vi "TEST_TestContoller.vi"() -> ()   [LabVIEW 2024]
uses:
  Control Definitions/Def_PumpSpeed.ctl
  Control Definitions/DEF_CalConstants.ctl
  Control Definitions/DEF_PumpCtlRefs.ctl
  Control Definitions/Def CalTable.ctl
  Control Definitions/Def CalCoef.ctl
  Control Definitions/Def_LevelCalCoef.ctl
  Control Definitions/Def_Status18v7.ctl
  Control Definitions/DEF_TestInfo.ctl
  Control Definitions/Def TestState.ctl
  Control Definitions/Registry Keys.ctl
  Control Definitions/Def Results3.ctl
  Control Definitions/Def_ATPStatus.ctl
  Control Definitions/Global 2.vi
  Control Definitions/Global 1.vi
panel:
  out "TEST State Out":T1
  in  "Sim":bool=TRUE
  out "Test Info":T2={"Job Number"="", "Unit Number"="", "Serial Number"="", "Technician Name"="", "Calibration Date"="Cal Date", "Calibrator"="Cal by", "Calibration Slope"="M", "Calibration Offset"="B", "Config File Name"="Cal Date"}
  out "Pump Out":T4
  out "Cal Coef":T5={"Level"={"M"=-0.9990777034816695, "B"=9.617362923679963, "Mc"=-1.0009231479344565, "Bc"=9.626241172397878, "LMe"=7.844}, "Dataq Ch"=[{"B"=-0.34241100677002123, "M"=175.4094780519764}, {"B"=-0.7865736704446391, "M"=174.89102005231038}]}
  in  "Default Cal Table":T7={"Level"={"LSf"=2.6, "LMf"=3.511, "LKf"=6.112, "LMe"=7.844, "LKe"=1.775, "LSe"=8.0}, "DataQ CH"=[{"RqLA"=0.577, "RmLA"=102.9, "RqHA"=5.052, "RmHA"=904.4}, {"RqLA"=0.577, "RmLA"=101.1, "RqHA"=5.116, "RmHA"=903.4}]}
  in  "End Prog":bool=TRUE
  out "Test Index Out":i32
  out "PumpCtlRef out":T8
  out "Reg Cal Constants":T9={"Measure High"="", "Laser High"="", "Measure Low"="", "Laser Low"="", "Cal Name"="", "Cal Date"="9/24/2024 9:21:12 AM", "Empty Inches"=8.0, "Full Inches"=2.6, "Valid"=FALSE}
  in  "Pump Speed":T10
  in  "SimPV":bool
  out "Root Path":path=path "C:/AllenProjects/PWC-OLS"
  out "Time(ms)":dbl=1249.4499999994114
  out "Level":bool=TRUE
  out "DataQ":bool=TRUE
  in  "ChA":dbl(slide)=24.489795918367346 scale=0.0..1200.0
  in  "ChB":dbl(slide)=36.73469387755102 scale=0.0..1200.0
  in  "ChB +100":bool
  in  "ChA +100":bool
  in  "Check":bool
  out "Laser (raw)":dbl=1.9040000438690186 format="%#_4g"
  in  "DUT":i16=1
  in  "Pump JOG":bool=TRUE
  in  "Run Test":bool
  in  "Normal":cluster{u32, u32}[](array[cluster])=[{16711680, 1244948}]
  out "Level \nStatus":bool=TRUE
  out "DataQ\nStatus":bool=TRUE
  in  "Level SP":dbl(slide)=8.0 scale=8.5..2.0
  in  "Level PV":dbl(slide)=7.715118932422306 scale=8.5..2.0
  out "Level":dbl=7.715118932422306 format="%.3f"
  in  "Drain":bool
  in  "Fill":bool
  out "TEST Name":string="OLR001--cal"
  out "Time Stamp":timestamp=timestamp(3810639016.2712703 s since 1904-01-01)
  in  "stop":bool
  out "ChB Ohms":dbl=100.0340857774357 format="%.1f"
  out "ChA Ohms":dbl=100.79497115454612 format="%.1f"
  # "Calibration & Scaling Table\n               Tank         Key          Ref\n               Scale        Level        Measure\nEmpty\n\n\nFull"
  # "8.0      1.7752      7.844\n\n2.6      6.112        3.511"
  # "CHA             Resistance     Fill     Resistance   Drain"
  # "CHB           Resistance     Fill     Resistance   Drain"
  # "Simulated Resistor In"
  # "PUMP"
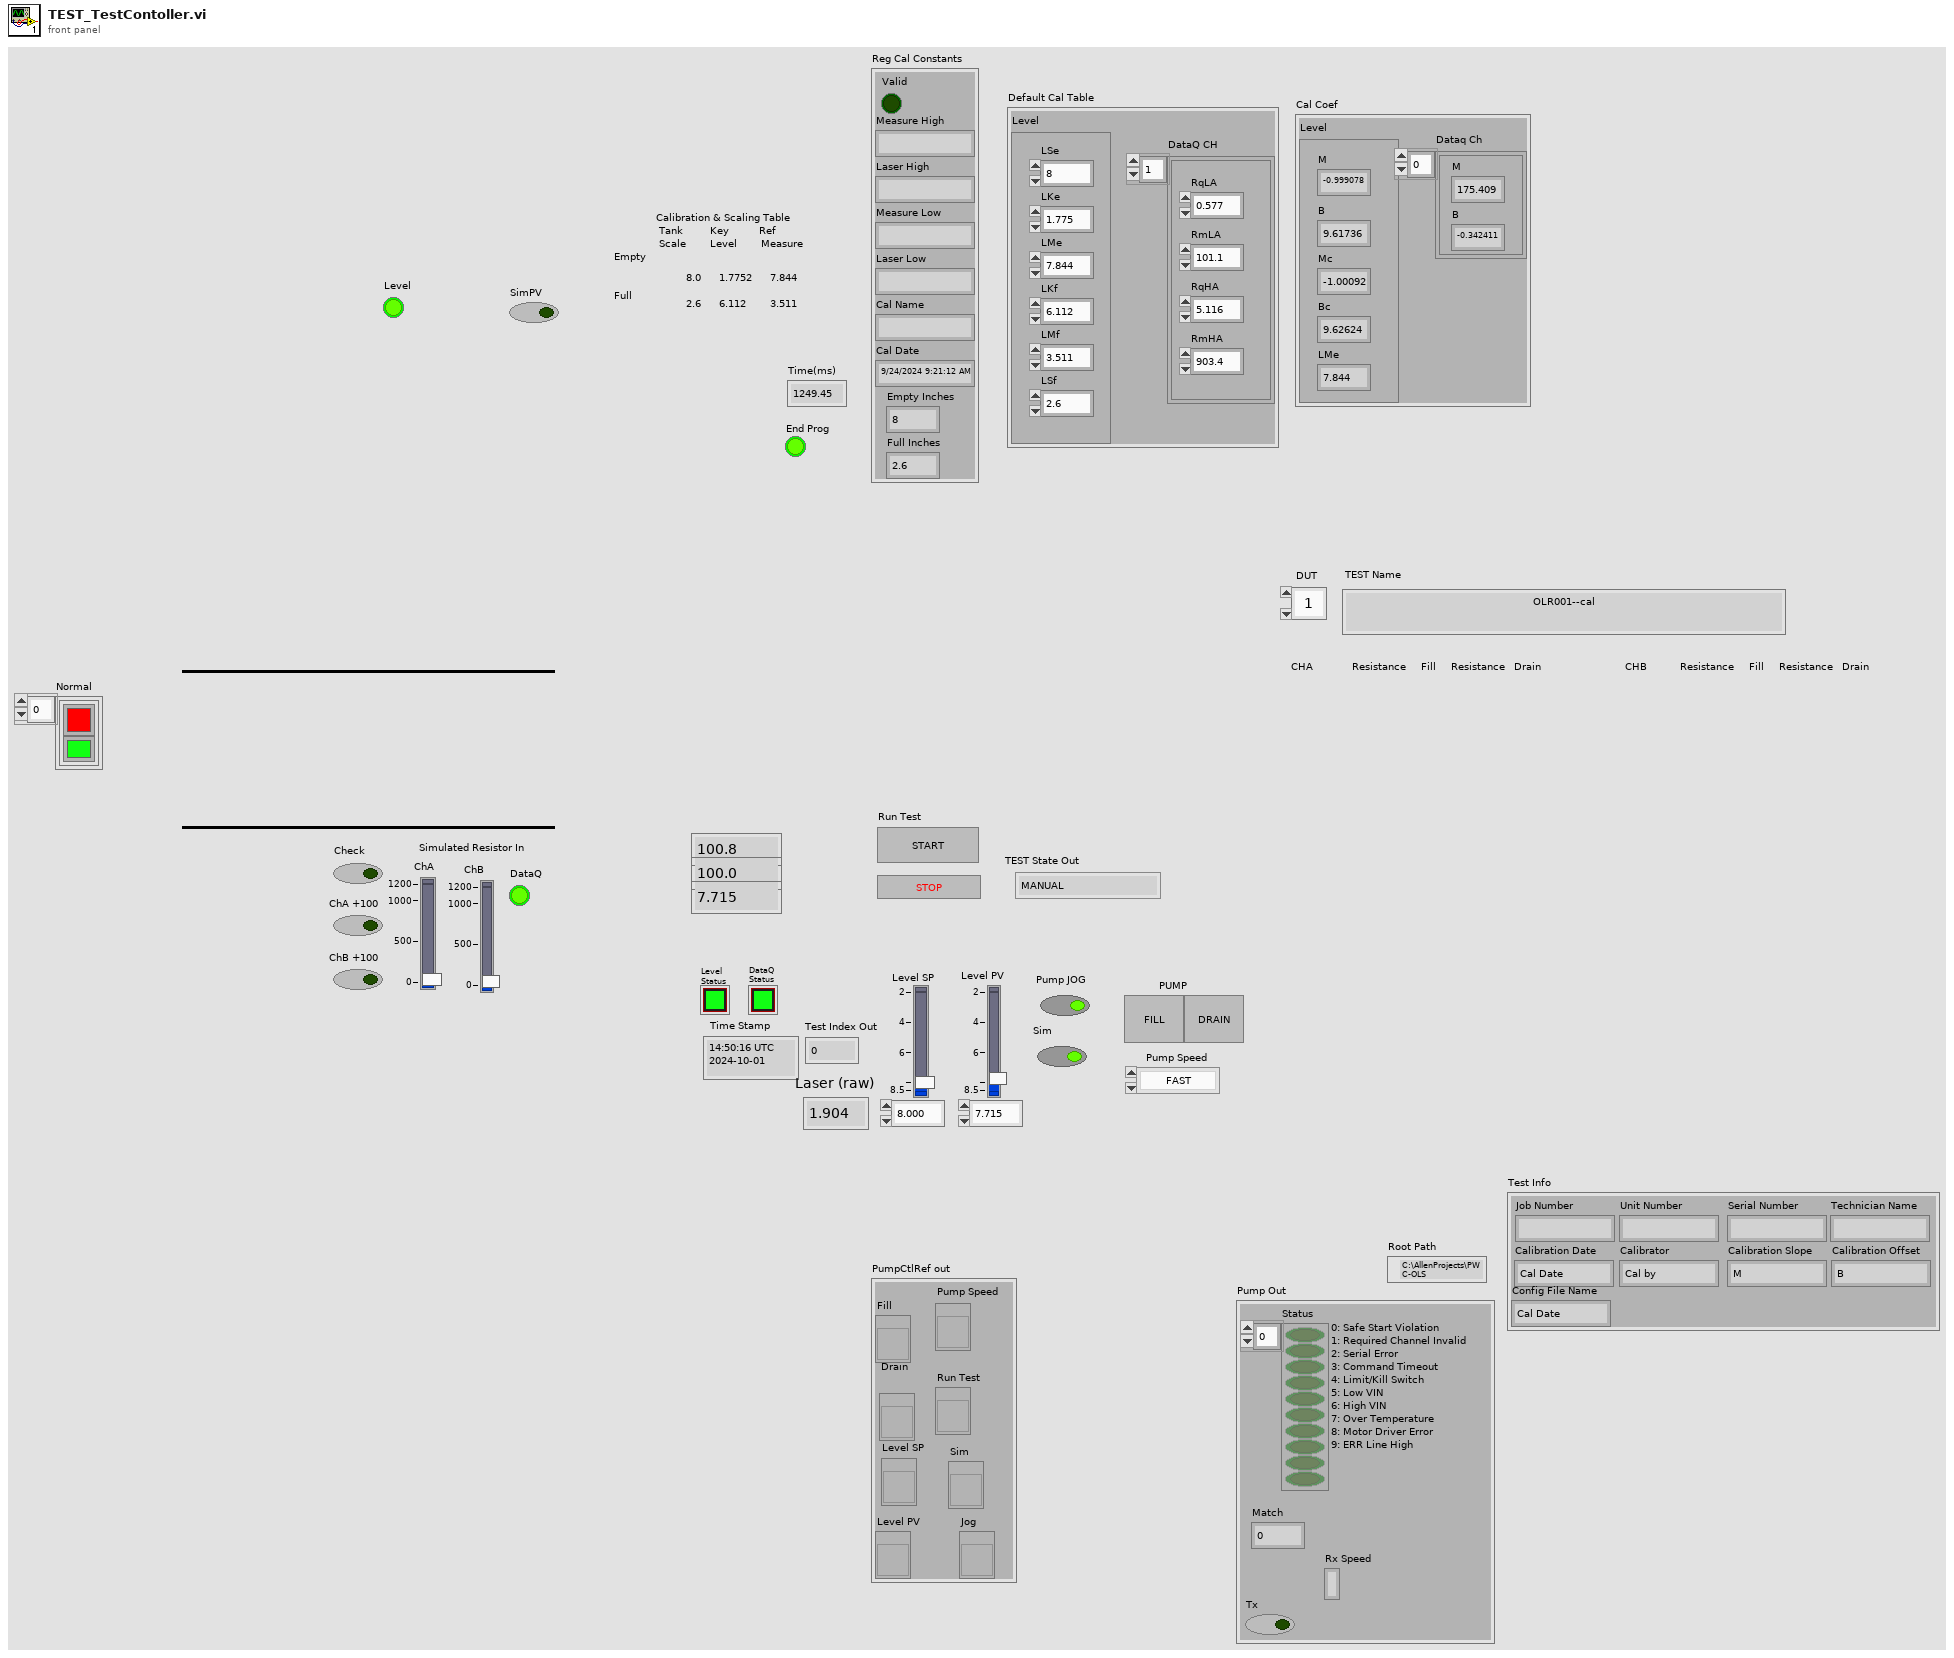
[diagram p1: front panel]
types:
  T1 = typedef "Def TestState.ctl" = enum16{"MANUAL", "Start", "Pre-Fill", "Pre-Fill Measure", "Pre-Drain", "Pre-Drain Measure", "Init-Record", "Load Fill Spec", "Filling Hi", "Wait1", "Record Fill", "Load Drain Spec", "Draining Lo", "Wait2", "Record Drain", "Empty", "Done"}
  T2 = typedef "DEF_TestInfo.ctl" = cluster{"Job Number":string, "Unit Number":string, "Serial Number":string, "Technician Name":string, "Calibration Date":string, "Calibrator":string, "Calibration Slope":string, "Calibration Offset":string, "Config File Name":string}
  T3 = typedef "Def_Status18v7.ctl" = bool[]
  T4 = cluster{"Status":T3, "Match":i32, "Rx Speed":string, "Tx":bool}
  T5 = typedef "Def CalCoef.ctl" = cluster{"Level":T6, "Dataq Ch":cluster{"B":dbl, "M":dbl}[]}
  T6 = typedef "Def_LevelCalCoef.ctl" = cluster{"M":dbl, "B":dbl, "Mc":dbl, "Bc":dbl, "LMe":dbl}
  T7 = typedef "Def CalTable.ctl" = cluster{"Level":cluster{"LSf":dbl, "LMf":dbl, "LKf":dbl, "LMe":dbl, "LKe":dbl, "LSe":dbl}, "DataQ CH":cluster{"RqLA":dbl, "RmLA":dbl, "RqHA":dbl, "RmHA":dbl}[]}
  T8 = typedef "DEF_PumpCtlRefs.ctl" = cluster{"Fill ":refnum<vi>, "Drain":refnum<vi>, "Level PV":refnum<vi>, "Pump Speed":refnum<vi>, "Run Test":refnum<vi>, "Sim":refnum<vi>, "Jog":refnum<vi>, "Level SP":refnum<vi>}
  T9 = typedef "DEF_CalConstants.ctl" = cluster{"Measure High":string, "Laser High":string, "Measure Low":string, "Laser Low":string, "Cal Name":string, "Cal Date":string, "Empty Inches":dbl, "Full Inches":dbl, "Valid":bool}
  T10 = typedef "Def_PumpSpeed.ctl" = enum16{"FAST", "SLOW", "CREEP", "STOP"}
  T11 = typedef "DEF_DataqParams.ctl" = cluster{"Visa Name":string, "Num Chan":i32, "Cal Coef":cluster{"M":dbl, "B":dbl}[], "Scale ":i32, "Cal Date":string, "Cal Technicain":string}
  T12 = typedef "DEF_18v7DriverInputs.ctl" = cluster{"Fill!Drain":bool, "Speed":i16, "Send Msg":bool, "Write Buf":string}
  T13 = typedef "Registry Keys.ctl" = enum16{"Report Files Key", "Config Files Key"}
  T14 = cluster{"Level \nStatus":refnum<vi>, "DataQ\nStatus":refnum<vi>}
  T15 = typedef "DEF_FullConfig.ctl" = cluster{"Bench Params":T16, "Test Params":dbl[][], "Pump Params":T17, "DataQ Params":T11, "Pump Control Ref":T8, "Bench Status":T18}
  T16 = typedef "DEF_BenchParams.ctl" = cluster{"Relative Root Name":string, "Values":cluster{"Step Levels":dbl, "Resistor Tolerence":dbl, "Sample Rate":dbl, "Resistor":dbl, "Wait Time":dbl}, "Report Template path":path, "Test Type":string, "Config File Name":string, "Config 2 Use":string, "Skip Pre Lube":bool}
  T17 = typedef "DEF_PumpParams.ctl" = cluster{"Empty Inches":dbl, "Full Inches":dbl, "RNG_SLOW":dbl, "RNG_CREEP":dbl, "RNG_STOP ":dbl, "VISA resource name":refnum<visa-resource-name>, "SPD_SLOW":i32, "SPD_CREEP":i32, "SPD_FAST":i32, "Zero template":path, "zero  Settle sec":i32, "Laser Slope":sgl, "Laser Offset":sgl, "Sim Fill Rate":sgl, "Cal Date":string, "Cal Technician":string}
  T18 = typedef "DEF_BenchStatus.ctl" = cluster{"Pump Status":refnum<vi>, "Instrumnet\n Status":refnum<vi>}
  T19 = typedef "Def Results3.ctl" = cluster{"Fill":dbl, "Status":T20, "Resistor":dbl, "Drain":dbl, "Resistor 2":dbl}
  T20 = typedef "Def_ATPStatus.ctl" = i16
  T21 = enum16{"MANUAL", "Start", "Filling", "FULL", "Draining", "EMPTY", "Done"}
  T22 = typedef "DEF_LevelOut.ctl" = cluster{"Laser ":cluster{"Raw":sgl, "Scaled":dbl}, "Level PV":dbl, "Fill":bool, "Drain":bool}
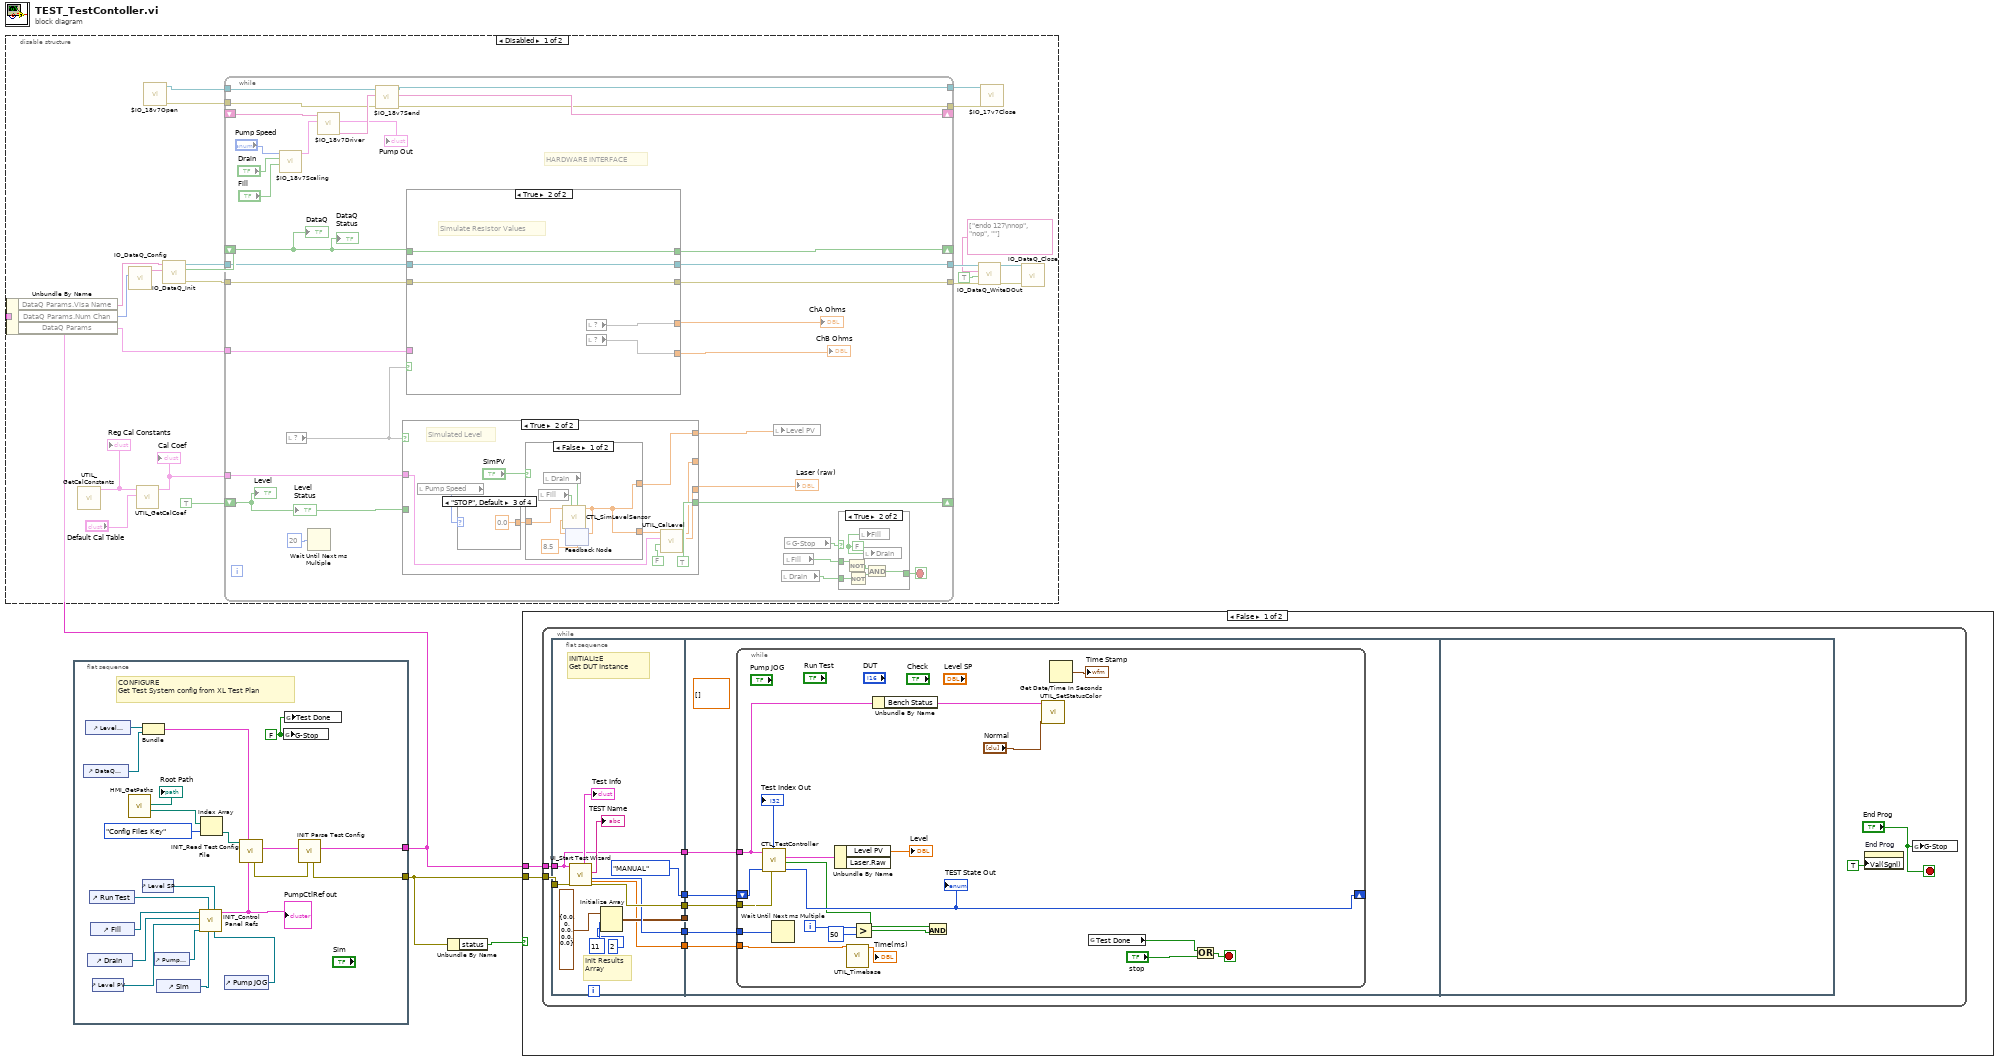
[diagram p0: block diagram]
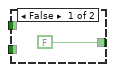
[diagram p2: hidden frame]
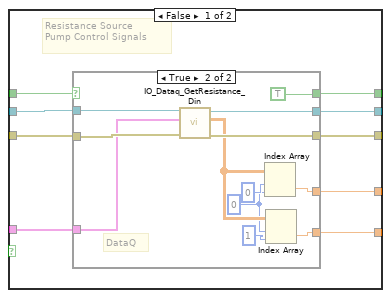
[diagram p3: hidden frame]
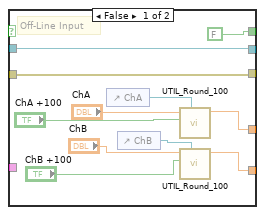
[diagram p4: hidden frame]
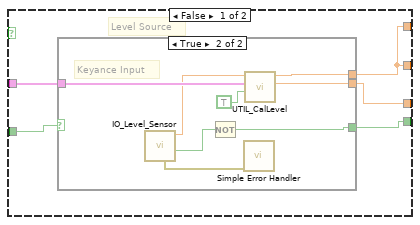
[diagram p5: hidden frame]
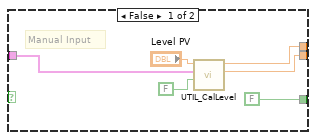
[diagram p6: hidden frame]
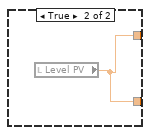
[diagram p7: hidden frame]
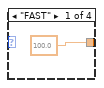
[diagram p8: hidden frame]
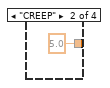
[diagram p9: hidden frame]
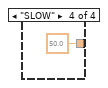
[diagram p10: hidden frame]
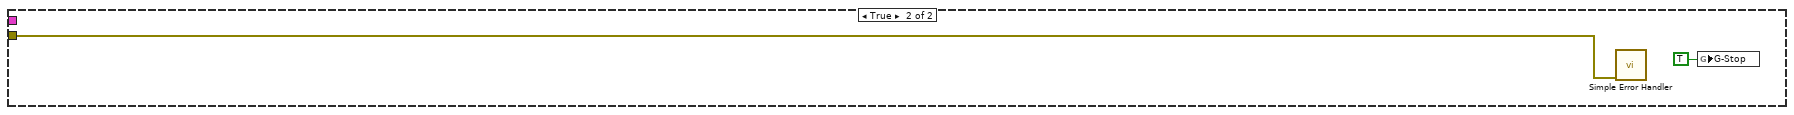
[diagram p12: hidden frame]
diagram:
  n1 = disable-structure shown="Disabled" {
    disable-tunnel: w1 -> [w4 _]
    frame Disabled {
      n2 = Unbundle By Name(w4) -> ("DataQ Params.Visa Name"=w6:string, "DataQ Params.Num Chan"=w7:i32, "DataQ Params"=w5:T11)
      n3 = call "UTIL_GetCalConstants.vi"() -> ("Cal Constants"=w14:T9)  [unwired: 10 in, 1 out]
      "Reg Cal Constants" <- w14
      n4 = call "IO_DataQ_Config.vi"("Num Chan"=w7) -> ("Init Message"=w25:string[])  [unwired: 10 in]
      n5 = call "UTIL_GetCalCoef.vi"("Cal Table"="Default Cal Table", "Cal Constants"=w14) -> ("Cal Coef"=w12:T5)  [unwired: 9 in]
      "Cal Coef" <- w12
      n6 = call "$IO_18v7Open.vi"() -> ("error out"=w11:errorcluster, "VISA Refnum out"=w10:refnum<visa-resource-name>)  [unwired: 10 in]
      n7 = call "IO_DataQ_Init.vi"("Command\nList"=w25, "RunTime VISA name"=w6) -> ("error out"=w23:errorcluster, "Connected?"=w22:bool, "VISA resource name out"=w24:refnum<visa-resource-name>)  [unwired: 7 in]
      n8 = while {
        shift-right: [w54] -> _
        shift-left: TRUE ("Pump \nStatus") -> [w41]
        tunnel: w24 -> [w53]
        tunnel: w23 -> [w52]
        tunnel: [w50] -> w20
        tunnel: [w51] -> w18
        shift-right: [w49] -> _
        shift-left: w22 -> [w48]
        tunnel: w12 -> [w26]
        shift-right: [w39] -> _
        shift-left: _ -> [w38]
        tunnel: w11 -> [w32]
        tunnel: w10 -> [w31]
        tunnel: [w30] -> w9
        tunnel: [w29] -> w8
        tunnel: w5 -> [w27]
        stop <- w45 stop-if-true
        # "HARDWARE INTERFACE"
        n9 = call "$IO_18v7Scaling.vi"("Drain"="Fill", "Fill"="Drain", "Pump Speed"="Pump Speed") -> ("Driver Signals"=w34:T12)  [unwired: 7 in, 1 out]
        n10 = local read item#-1() -> (w47)
        n11 = Wait Until Next ms Multiple(millisecond multiple=u32 20) -> ()  [unwired: 1 out]
        n12 = call "$IO_18v7Driver.vi"("Inputs"=w34, "Reply In"=w38) -> ("Tx Buf Out"=w33:string, "Outputs"=→"Pump Out":T4)  [unwired: 8 in]
        n13 = call "$IO_18v7Send.vi"("error in (no error)"=w32, "Tx Buf Out"=w33, "VISA Refnum in"=w31) -> ("error out"=w29:errorcluster, "read buffer"=w39:string, "VISA Refnum out"=w30:refnum<visa-resource-name>)  [unwired: 6 in]
        n14 = case shown="True" w47 {
          tunnel: [w102 w127] -> _
          tunnel: [w106 w129] -> w55
          tunnel: [w103 TRUE] -> w54
          tunnel: w41 -> [w105 _]
          tunnel: w26 -> [w104 w122]
          tunnel: [w102 w121] -> w40
          frame False {
            # "Level Source"
            n15 = case shown="True" w105 {
              tunnel: [w110 w113] -> w102
              tunnel: [w109 w118] -> w106
              tunnel: [FALSE ("status") w117] -> w103
              tunnel: w104 -> [w111 w119]
              frame False {
                # "Manual Input"
                n16 = call "UTIL_CalLevel.vi"("Key is In?"=FALSE, "Cal Coef"=w111, "Input"="Level PV") -> ("PVc"=w109:dbl, "PVs"=w110:dbl)  [unwired: 7 in]
              }
              frame True {
                # "Keyance Input"
                n17 = call "IO_Level_Sensor.vi"() -> ("status"=w115:bool, "PV (raw)"=w116:dbl, "error OUT"=w114:errorcluster)  [unwired: 9 in]
                n18 = Not(x=w115) -> (.not. x?=w117:bool)
                n19 = call <vilib>:"Simple Error Handler.vi"("error in (no error)"=w114) -> ()  [unwired: 4 in, 5 out]
                n20 = call "UTIL_CalLevel.vi"("Key is In?"=TRUE, "Cal Coef"=w119, "Input"=w116) -> ("PVc"=w118:dbl, "PVs"=w113:dbl)  [unwired: 7 in]
              }
            }
          }
          frame True {
            # "Simulated Level"
            n21 = local read "Pump Speed"() -> (w125:T10)
            n22 = case shown="\"STOP\", Default" w125 {
              tunnel: [100.0 ("Ctl Sig") 5.0 ("Ctl Sig") 0.0 ("Ctl Sig") 50.0 ("Ctl Sig")] -> w126
              frame "FAST" {
              }
              frame "CREEP" {
              }
              frame "STOP", Default {
              }
              frame "SLOW" {
              }
            }
            n23 = case shown="False" "SimPV" {
              tunnel: w126 -> [w135 _]
              tunnel: [w131 w137] -> w124
              tunnel: [w131 w137] -> w121
              frame False {
                n24 = local read "Fill"() -> (w136:bool)
                n25 = local read "Drain"() -> (w132:bool)
                n26 = feedback #1(8.5 ("PV Level Inch")) -> (w133:dbl)
                n27 = call "CTL_SimLevelSensor.vi"("Drain IN"=w132, "Fill IN"=w136, "Level PV in"=w133, "Pump Speed"=w135) -> ("PV Level Inch"=w131:dbl)  [unwired: 7 in]
                n28 = feedback-in #1(w131) -> ()
              }
              frame True {
                n29 = local read "Level PV"() -> (w137:dbl)
              }
            }
            n30 = call "UTIL_CalLevel.vi"("Key is In?"=FALSE, "Cal Coef"=w122, "Input"=w124) -> ("PVc"=w129:dbl, "PVs"=w127:dbl)  [unwired: 7 in]
          }
        }
        "Laser (raw)" <- w55
        n31 = case shown="True" w47 {
          tunnel: [w73 w98] -> w56
          tunnel: [w72 w97] -> w42
          tunnel: w53 -> [w66 w100]
          tunnel: w52 -> [w67 w99]
          tunnel: [w71 w99] -> w51
          tunnel: [w70 w100] -> w50
          tunnel: [w69 w101] -> w49
          tunnel: w48 -> [w68 w101]
          tunnel: w27 -> [w65 _]
          frame False {
            # "Resistance Source\nPump Control Signals"
            n32 = case shown="True" w68 {
              tunnel: [w77 w93] -> w73
              tunnel: [w78 w90] -> w72
              tunnel: [w79 w96] -> w70
              tunnel: [w80 w95] -> w71
              tunnel: [FALSE TRUE] -> w69
              tunnel: w67 -> [w80 w86]
              tunnel: w66 -> [w79 w87]
              tunnel: w65 -> [_ w85]
              frame False {
                # "Off-Line Input"
                n33 = control-ref of="ChA"() -> (w76:refnum<vi>)
                n34 = control-ref of="ChB"() -> (w74:refnum<vi>)
                n35 = call "UTIL_Round_100.vi"("Num Refnum"=w76, "100"="ChA +100", "IN"="ChA") -> ("OUT"=w78:dbl)  [unwired: 8 in]
                n36 = call "UTIL_Round_100.vi"("Num Refnum"=w74, "100"="ChB +100", "IN"="ChB") -> ("OUT"=w77:dbl)  [unwired: 8 in]
              }
              frame True {
                w89 = 0 ("disabled index (col)")
                # "DataQ"
                n37 = call "IO_Dataq_GetResistance_Din.vi"("error in (no error)"=w86, "Dataq Params"=w85, "VISA Refnum in"=w87) -> ("error out"=w95:errorcluster, "Analog"=w91:dbl[][], "VISA Refnum out"=w96:refnum<visa-resource-name>)  [unwired: 5 in, 1 out]
                n38 = Index Array(array=w91, index (row)=0 ("index"), index (col)=w89) -> (element=w90:dbl)
                n39 = Index Array(array=w91, index (row)=w89, index (col)=1 ("index")) -> (element=w93:dbl)
              }
            }
          }
          frame True {
            # "Simulate Resistor Values"
            n40 = local read item#-1() -> (w97)
            n41 = local read item#-1() -> (w98)
          }
        }
        "ChA Ohms" <- w42
        "ChB Ohms" <- w56
        n42 = local write "Level PV"(w40) -> ()
        n43 = local read "Drain"() -> (w43:bool)
        n44 = local read "Fill"() -> (w44:bool)
        n45 = global read "Global 1.vi" "G-Stop"() -> (w46:bool)
        n46 = case shown="True" w46 {
          tunnel: [FALSE w60] -> w45
          tunnel: w44 -> [_ w62]
          tunnel: w43 -> [_ w59]
          frame False {
          }
          frame True {
            w64 = FALSE
            n47 = Not(x=w62) -> (.not. x?=w63:bool)
            n48 = Not(x=w59) -> (.not. x?=w61:bool)
            n49 = local write "Fill"(w64) -> ()
            n50 = local write "Drain"(w64) -> ()
            n51 = And(x=w63, y=w61) -> (x .and. y?=w60:bool)
          }
        }
        "DataQ\nStatus" <- w48
        "Level \nStatus" <- w41
        "DataQ" <- w48
        "Level" <- w41
      }
      n52 = call "IO_DataQ_WriteDOut.vi"("error in (no error)"=w18, "Msg Active"=TRUE, "Message"=string[] ["endo 127\nnop", "nop", ""], "VISA Refnum in"=w20) -> ("error out"=w17:errorcluster, "VISA Refnum out"=w19:refnum<visa-resource-name>)  [unwired: 6 in]
      n53 = call "$IO_17v7Close.vi"("error in (no error)"=w8, "VISA Refnum in"=w9) -> ()  [unwired: 10 in]
      n54 = call "IO_DataQ_Close.vi"("error in"=w17, "VISA resource name"=w19) -> ()  [unwired: 10 in]
    }
    frame Enabled {
    }
  }
  n55 = flat-sequence {
    tunnel: [w144] -> w2
    tunnel: [w157] -> w1
    frame #0 {
      w153 = FALSE ("G-Stop")
      # "CONFIGURE\nGet Test System config from XL Test Plan"
      n56 = control-ref of="DataQ\nStatus"() -> (w155:refnum<vi>)
      n57 = control-ref of="Level \nStatus"() -> (w161:refnum<vi>)
      n58 = control-ref of="Drain"() -> (w162:refnum<vi>)
      n59 = control-ref of="Run Test"() -> (w158:refnum<vi>)
      n60 = control-ref of="Fill"() -> (w159:refnum<vi>)
      n61 = control-ref of="Level PV"() -> (w160:refnum<vi>)
      n62 = call "HMI_GetPaths.vi"() -> ("Default Paths"=w149:path[], "Root Path"=→"Root Path":path)  [unwired: 10 in]
      n63 = Bundle("Level \nStatus"=w161, "DataQ\nStatus"=w155) -> (w147:T14)  [unwired: 1 in]
      n64 = control-ref of="Level SP"() -> (w154:refnum<vi>)
      n65 = control-ref of="Pump Speed"() -> (w151:refnum<vi>)
      n66 = control-ref of="Sim"() -> (w142:refnum<vi>)
      n67 = Index Array(array=w149, index=Registry_Keys."Config Files Key" ("Reg Key")) -> (element=w148:path)
      n68 = control-ref of="Pump JOG"() -> (w156:refnum<vi>)
      n69 = call "INIT_Control Panel Refs.vi"("Jog"=w156, "Level SP"=w154, "Sim"=w142, "Run Test"=w158, "Pump Speed"=w151, "Level PV"=w160, "Drain"=w162, "Fill"=w159) -> ("PumpCtlRef out"=w146:T8)  [unwired: 3 in]
      "PumpCtlRef out" <- w146
      n70 = call "INIT_Read Test Config File.vi"("Pump Control Ref"=w146, "Bench Status"=w147, "Path"=w148) -> ("FullConfig"=w143:T15, "error out"=w145:errorcluster)  [unwired: 7 in]
      n71 = global write "Global 1.vi" "G-Stop"(w153) -> ()
      n72 = global write "Global 2.vi" "Test Done"(w153) -> ()
      n73 = call "INIT Parse Test Config.vi"("error in"=w145, "Full Config In"=w143) -> ("Full Config Out"=w157:T15, "error out"=w144:errorcluster)  [unwired: 8 in]
    }
  }
  n74 = Unbundle By Name(w2) -> ("status"=w3:bool)
  n75 = case shown="False" w3 {
    tunnel: w2 -> [w164 w212]
    tunnel: w1 -> [w163 _]
    frame False {
      n76 = while {
        tunnel: w164 -> [w172]
        tunnel: w163 -> [w166]
        stop <- "End Prog" stop-if-true
        n77 = flat-sequence {
          tunnel: [w184] -> w174
          tunnel: [w185] -> w173
          tunnel: w172 -> [w186]
          tunnel: [w175] -> w171
          tunnel: [T21."MANUAL" ("TEST STATUS Out")] -> w170
          tunnel: [w180] -> w169
          tunnel: [w179] -> w168
          tunnel: w166 -> [w175]
          tunnel: w174 -> [w190]
          tunnel: w173 -> [w191]
          tunnel: w171 -> [w187]
          tunnel: w170 -> [w188]
          tunnel: w169 -> [_]
          tunnel: w168 -> [w189]
          frame #0 {
            # "Init Results\nArray"
            # "INITIALIzE\nGet DUT Instance"
            n78 = call "UI_Start Test Wizard.vi"("error in (no error)"=w186, "Full Config"=w175) -> ("error out"=w185:errorcluster, "Time Base mS"=w184:i32, "Title"=→"TEST Name":string, "Sample Rate"=w179:dbl, "Test Info"=→"Test Info":T2)  [unwired: 3 in]
            n79 = Initialize Array(T19 {"Fill"=0.0, "Status"=0, "Resistor"=0.0, "Drain"=0.0, "Resistor 2"=0.0} ("Cluster 2"), 11 ("dimension size"), 2 ("dimension size")) -> (w180:T19[][])
          }
          frame #1 {
            (unwired) dbl[][] [] ("Array")
            n80 = while {
              tunnel: w190 -> [w210]
              tunnel: w191 -> [w204]
              tunnel: w189 -> [w203]
              shift-right: [w198] -> _
              shift-left: w188 -> [w197]
              tunnel: w187 -> [w194]
              i -> [w202]
              stop <- w207 stop-if-true
              n81 = call "CTL_TestController.vi"("error in (no error)"=w204, "TEST State In"=w197, "FullConfig"=w194) -> ("TEST State Out"=w198:T1, "Enable"=w196:bool, "Level Out"=w193:T22, "Test Index Out"=→"Test Index Out":i32)  [unwired: 3 in, 2 out]
              "TEST State Out" <- w198
              n82 = Wait Until Next ms Multiple(millisecond multiple=w210) -> ()  [unwired: 1 out]
              n83 = Unbundle By Name(w193) -> ("Level PV"=→"Level":dbl)  [unwired: 1 out]
              n84 = call "UTIL_Timebase.vi"("Sample Rate"=w203) -> ("Time(ms)"=→"Time(ms)":dbl)  [unwired: 10 in]
              n85 = Greater?(x=w202, y=50) -> (0:w200:bool)
              n86 = Unbundle By Name(w194) -> ("Bench Status"=w208:T18)
              n87 = And(x=w196, y=w200) -> ()  [unwired: 1 out]
              n88 = call "UTIL_SetStatusColor.vi"("Colors [4] in"="Normal", "Bench Status"=w208) -> ()  [unwired: 10 in]
              n89 = Get Date/Time In Seconds() -> (seconds since 1Jan1904=→"Time Stamp":timestamp)
              n90 = global read "Global 2.vi" "Test Done"() -> (w205:bool)
              n91 = Or(x=w205, y="stop") -> (x .or. y?=w207:bool)
            }
          }
          frame #2 {
          }
        }
        n92 = property on="End Prog" class="Bool (strict)"("Val(Sgnl)"=TRUE ("End Prog")) -> ()  [unwired: 2 in, 2 out]
        n93 = global write "Global 1.vi" "G-Stop"("End Prog") -> ()
      }
    }
    frame True {
      n94 = call <vilib>:"Simple Error Handler.vi"("error in (no error)"=w212) -> ()  [unwired: 4 in, 5 out]
      n95 = global write "Global 1.vi" "G-Stop"(TRUE ("G-Stop")) -> ()
    }
  }
